vi "Disabled.vi"(7 "Robot Mode":T2, 10 "Match Info":T1={"Autonomous Elapsed Seconds"=0.0, "TeleOp Elapsed Seconds"=0.0, "Disabled Elapsed Seconds"=0.0, "Visited Autonomous"=FALSE, "Visited TeleOp"=FALSE, "Visited Disabled"=FALSE, "Autonomous Settings"={"Autonomous Style"=enum."Independent", "VI Refnum"=refnum}}, 11 "Call Context":T3) -> ()   [LabVIEW 2011]
doc: "This VI is called each time a disabled packet is received from the DS. It is often used to prepare for the next robot mode, to calibrate sensors, etc."
uses:
  <vilib>/Rock Robotics/WPI/DriverStation/WPI_DriverStationDerivedRobotMode.ctl
  <vilib>/Rock Robotics/WPI/DriverStation/WPI_DriverStationRobotMode.ctl
  <vilib>/Rock Robotics/WPI/DriverStation/WPI_DriverStationMatch Info.ctl
  Robot Global Data.vi
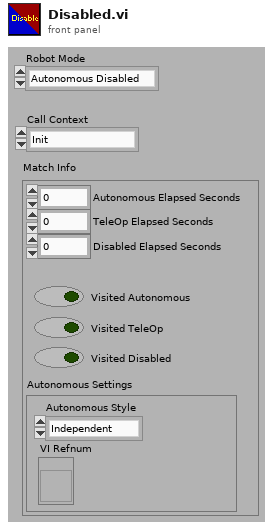
[diagram p1: front panel]
types:
  T1 = typedef "WPI_DriverStationMatch Info.ctl" = cluster{"Autonomous Elapsed Seconds":dbl, "TeleOp Elapsed Seconds":dbl, "Disabled Elapsed Seconds":dbl, "Visited Autonomous":bool, "Visited TeleOp":bool, "Visited Disabled":bool, "Autonomous Settings":cluster{"Autonomous Style":enum16{"Iterative", "Independent"}, "VI Refnum":refnum<vi>}}
  T2 = typedef "WPI_DriverStationRobotMode.ctl" = enum16{"Autonomous Disabled", "Autonomous Enabled", "Teleop Disabled", "Teleop Enabled", "Timeout", "Finish"}
  T3 = typedef "WPI_DriverStationDerivedRobotMode.ctl" = enum16{"Init", "Execute", "Stop"}
  T4 = typedef "WPI_MotorControlDeviceRef.ctl" = cluster{"DeviceStatus":errorcluster, "Type":enum16{"PWM", "CAN"}, "PWM":cluster{"Digital Module":T5, "PWM Channel":T6, "DeadBand":T7}, "CAN":cluster{"Device Number":u8, "Control Mode":T8, "Semaphore":T9, "Max Vout":dbl}, "Invert":bool, "TransformRef":T10, "InvTransformRef":T10}
  T5 = typedef "FPGA_TypedefDigitalModule.ctl" = enum16{"Digital Module 1", "Digital Module 2"}
  T6 = typedef "FPGA_DIOPWMChannel.ctl" = enum8{"PWM 1", "PWM 2", "PWM 3", "PWM 4", "PWM 5", "PWM 6", "PWM 7", "PWM 8", "PWM 9", "PWM 10", "Invalid"}
  T7 = typedef "WPI_PWMDeadband.ctl" = cluster{"Name":string, "maxPositivePwm":i32, "minPositivePwm":i32, "centerPwm":i32, "maxNegativePwm":i32, "minNegativePwm":i32, "angularRange":u16}
  T8 = typedef "WPI_CANJaguar_ControlMode.ctl" = enum8{"Percent VBus", "Current", "Speed", "Position", "Voltage"}
  T9 = typedef "Semaphore RefNum" = refnum<k1>
  T10 = typedef "WPI_PWMTransform_ConPane.ctl" = refnum<vi>
  T11 = typedef "WPI_JoystickDevRef.ctl" = cluster{"Device":T12}
  T12 = typedef "WPI_JoystickDeviceEnum.ctl" = enum16{"USB 1", "USB 2", "USB 3", "USB 4", "Kinect 1", "Kinect 2"}
  T13 = typedef "WPI_JoystickButtonState.ctl" = cluster{"Button 1":bool, "Button 2":bool, "Button 3":bool, "Button 4":bool, "Button 5":bool, "Button 6":bool, "Button 7":bool, "Button 8":bool, "Button 9":bool, "Button 10":bool, "Button 11":bool, "Button 12":bool}
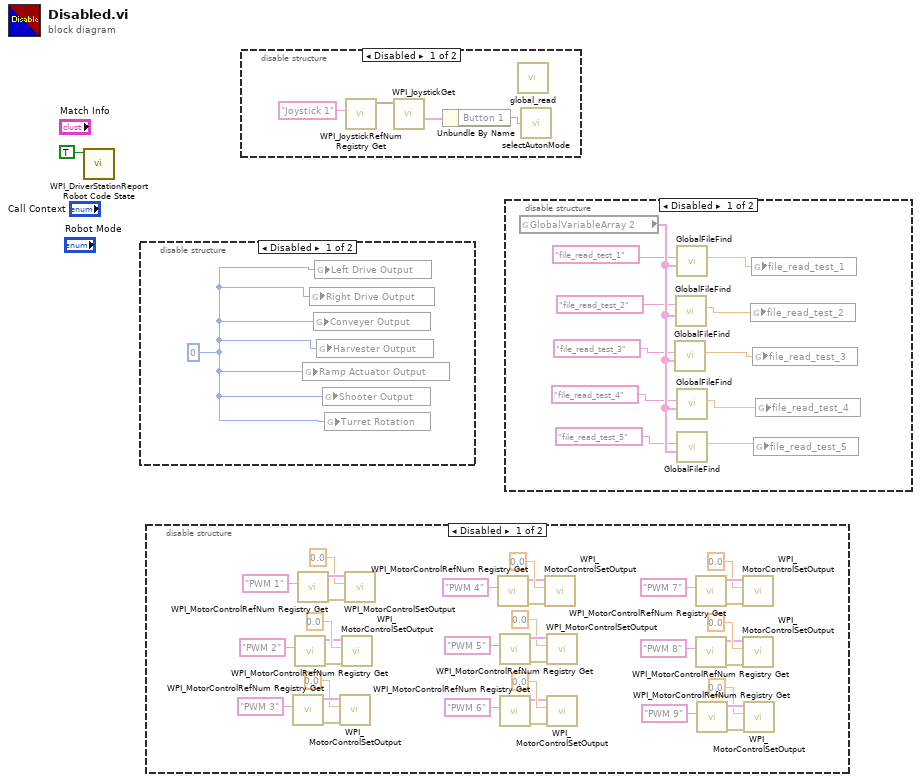
[diagram p0: block diagram]
diagram:
  n1 = call <vilib>:"WPI_DriverStationReport Robot Code State.vi"("Disabled"=TRUE ("Autonomous")) -> ()  [unwired: 10 in, 1 out]
  n2 = disable-structure shown="Disabled" {
    frame Disabled {
      w2 = 0
      n3 = global write "Robot Global Data.vi" "Ramp Actuator Output"(w2) -> ()
      n4 = global write "Robot Global Data.vi" "Right Drive Output"(w2) -> ()
      n5 = global write "Robot Global Data.vi" "Conveyer Output"(w2) -> ()
      n6 = global write "Robot Global Data.vi" "Left Drive Output"(w2) -> ()
      n7 = global write "Robot Global Data.vi" "Harvester Output"(w2) -> ()
      n8 = global write "Robot Global Data.vi" "Shooter Output"(w2) -> ()
      n9 = global write "Robot Global Data.vi" "Turret Rotation"(w2) -> ()
    }
    frame Enabled {
    }
  }
  n10 = disable-structure shown="Disabled" {
    frame Disabled {
      n11 = call <vilib>:"WPI_MotorControlRefNum Registry Get.vi"("refnum name"="PWM 3") -> ("error out"=w29:errorcluster, "MotorControlDevRef"=w30:T4)  [unwired: 9 in]
      n12 = call <vilib>:"WPI_MotorControlRefNum Registry Get.vi"("refnum name"="PWM 2") -> ("error out"=w32:errorcluster, "MotorControlDevRef"=w31:T4)  [unwired: 9 in]
      n13 = call <vilib>:"WPI_MotorControlRefNum Registry Get.vi"("refnum name"="PWM 1") -> ("error out"=w37:errorcluster, "MotorControlDevRef"=w38:T4)  [unwired: 9 in]
      n14 = call <vilib>:"WPI_MotorControlSetOutput.vi"("error in (no error)"=w29, "Output"=0.0, "MotorControlDevRef"=w30) -> ()  [unwired: 7 in, 2 out]
      n15 = call <vilib>:"WPI_MotorControlSetOutput.vi"("error in (no error)"=w32, "Output"=0.0, "MotorControlDevRef"=w31) -> ()  [unwired: 7 in, 2 out]
      n16 = call <vilib>:"WPI_MotorControlSetOutput.vi"("error in (no error)"=w37, "Output"=0.0, "MotorControlDevRef"=w38) -> ()  [unwired: 7 in, 2 out]
      n17 = call <vilib>:"WPI_MotorControlRefNum Registry Get.vi"("refnum name"="PWM 4") -> ("error out"=w24:errorcluster, "MotorControlDevRef"=w23:T4)  [unwired: 9 in]
      n18 = call <vilib>:"WPI_MotorControlRefNum Registry Get.vi"("refnum name"="PWM 5") -> ("error out"=w21:errorcluster, "MotorControlDevRef"=w22:T4)  [unwired: 9 in]
      n19 = call <vilib>:"WPI_MotorControlRefNum Registry Get.vi"("refnum name"="PWM 6") -> ("error out"=w16:errorcluster, "MotorControlDevRef"=w15:T4)  [unwired: 9 in]
      n20 = call <vilib>:"WPI_MotorControlSetOutput.vi"("error in (no error)"=w24, "Output"=0.0, "MotorControlDevRef"=w23) -> ()  [unwired: 7 in, 2 out]
      n21 = call <vilib>:"WPI_MotorControlSetOutput.vi"("error in (no error)"=w21, "Output"=0.0, "MotorControlDevRef"=w22) -> ()  [unwired: 7 in, 2 out]
      n22 = call <vilib>:"WPI_MotorControlSetOutput.vi"("error in (no error)"=w16, "Output"=0.0, "MotorControlDevRef"=w15) -> ()  [unwired: 7 in, 2 out]
      n23 = call <vilib>:"WPI_MotorControlRefNum Registry Get.vi"("refnum name"="PWM 7") -> ("error out"=w13:errorcluster, "MotorControlDevRef"=w14:T4)  [unwired: 9 in]
      n24 = call <vilib>:"WPI_MotorControlRefNum Registry Get.vi"("refnum name"="PWM 8") -> ("error out"=w8:errorcluster, "MotorControlDevRef"=w7:T4)  [unwired: 9 in]
      n25 = call <vilib>:"WPI_MotorControlRefNum Registry Get.vi"("refnum name"="PWM 9") -> ("error out"=w5:errorcluster, "MotorControlDevRef"=w6:T4)  [unwired: 9 in]
      n26 = call <vilib>:"WPI_MotorControlSetOutput.vi"("error in (no error)"=w13, "Output"=0.0, "MotorControlDevRef"=w14) -> ()  [unwired: 7 in, 2 out]
      n27 = call <vilib>:"WPI_MotorControlSetOutput.vi"("error in (no error)"=w8, "Output"=0.0, "MotorControlDevRef"=w7) -> ()  [unwired: 7 in, 2 out]
      n28 = call <vilib>:"WPI_MotorControlSetOutput.vi"("error in (no error)"=w5, "Output"=0.0, "MotorControlDevRef"=w6) -> ()  [unwired: 7 in, 2 out]
    }
    frame Enabled {
    }
  }
  n29 = disable-structure shown="Disabled" {
    frame Disabled {
      n30 = call <vilib>:"WPI_JoystickRefNum Registry Get.vi"("refnum name"="Joystick 1") -> ("JoystickDevRef"=w41:T11)  [unwired: 9 in, 1 out]
      n31 = call <vilib>:"WPI_JoystickGet.vi"("JoystickDevRef"=w41) -> ("Buttons"=w40:T13)  [unwired: 4 in, 2 out]
      n32 = Unbundle By Name(w40) -> ("Button 1"=w39:bool)
      n33 = call "global_read.vi"() -> ()  [unwired: 12 in]
      n34 = call "selectAutonMode.vi"("Joystick"=w39) -> ()  [unwired: 1 in]
    }
    frame Enabled {
    }
  }
  n35 = disable-structure shown="Disabled" {
    frame Disabled {
      n36 = global read "Robot Global Data.vi" "GlobalVariableArray 2"() -> (w53:cluster{"name":string, "va;":dbl}[])
      n37 = call "GlobalFileFind.vi"("GlobalVariableArray 2"=w53, "VariableNameLookup"="file_read_test_3") -> ("VariableValueOut"=w44:dbl)  [unwired: 9 in]
      n38 = call "GlobalFileFind.vi"("GlobalVariableArray 2"=w53, "VariableNameLookup"="file_read_test_2") -> ("VariableValueOut"=w43:dbl)  [unwired: 9 in]
      n39 = call "GlobalFileFind.vi"("GlobalVariableArray 2"=w53, "VariableNameLookup"="file_read_test_1") -> ("VariableValueOut"=w47:dbl)  [unwired: 9 in]
      n40 = call "GlobalFileFind.vi"("GlobalVariableArray 2"=w53, "VariableNameLookup"="file_read_test_4") -> ("VariableValueOut"=w45:dbl)  [unwired: 9 in]
      n41 = call "GlobalFileFind.vi"("GlobalVariableArray 2"=w53, "VariableNameLookup"="file_read_test_5") -> ("VariableValueOut"=w46:dbl)  [unwired: 9 in]
      n42 = global write "Robot Global Data.vi" "file_read_test_2"(w43) -> ()
      n43 = global write "Robot Global Data.vi" "file_read_test_1"(w47) -> ()
      n44 = global write "Robot Global Data.vi" "file_read_test_3"(w44) -> ()
      n45 = global write "Robot Global Data.vi" "file_read_test_5"(w46) -> ()
      n46 = global write "Robot Global Data.vi" "file_read_test_4"(w45) -> ()
    }
    frame Enabled {
    }
  }
